vi "getSerial.vi"(0 "Camera in":refnum<class "Camera.lvclass">, 11 "error in (no error)":errorcluster) -> (4 "Camera out":refnum<class "Camera.lvclass">, 6 "serial_number":u32, 15 "error out":errorcluster)   [LabVIEW 2019, in "Camera.lvclass"]
doc: "Gets the serial number of the connected camera."
uses:
  Camera.lvclass
  Camera.lvclass/Camera.ctl
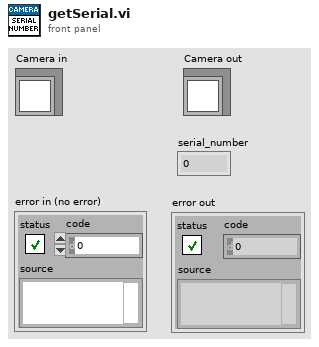
[diagram p1: front panel]
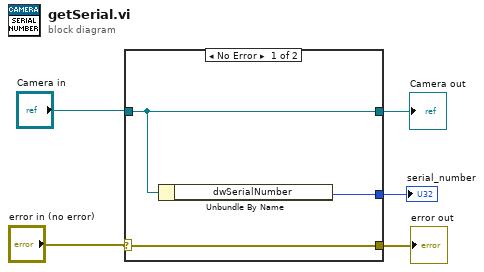
[diagram p0: block diagram]
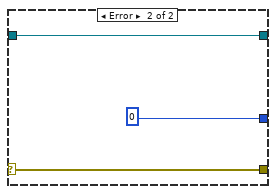
[diagram p2: hidden frame]
diagram:
  n1 = case shown="No Error" "error in (no error)" {
    selector: "error in (no error)" -> [w7 w11]
    tunnel: [w7 w11] -> w3
    tunnel: [w8 w10] -> w4
    tunnel: "Camera in" -> [w8 w10]
    tunnel: [w6 u32 0 ("dwErr")] -> w1
    frame No Error {
      n2 = Unbundle By Name(w8) -> ("dwSerialNumber"=w6:u32)
    }
    frame Error {
    }
  }
  "error out" <- w3
  "Camera out" <- w4
  "serial_number" <- w1
